vi "多参数标样核查对话框.vi"() -> (2 "确认":bool, 3 "输出参数":T1)   [LabVIEW 2016, in "斯坦道仪器.lvlib"]
panel:
  in  "浊度":bool
  in  "电导率":bool
  in  "pH":bool
  in  "DO":bool
  in  "水温":bool
  in  "组数":dbl=3.0
  in  "取消":bool
  in  "确定":bool
  # "请输入启动参数"
  # "保存组数"
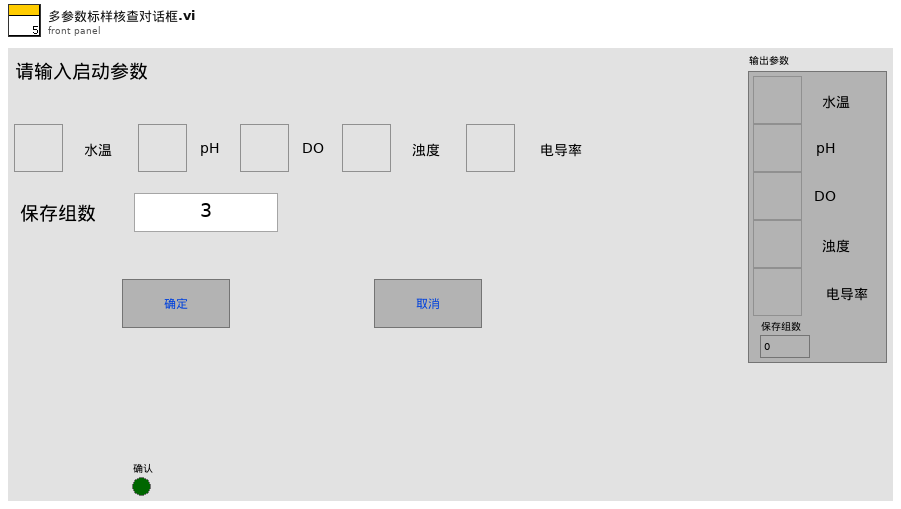
[diagram p1: front panel]
types:
  T1 = cluster{"水温":bool, "pH":bool, "DO":bool, "浊度":bool, "电导率":bool, "保存组数":dbl}
  T2 = cluster{"水温":bool, "pH":bool, "DO":bool, "浊度":bool, "电导率":bool, "组数":dbl}
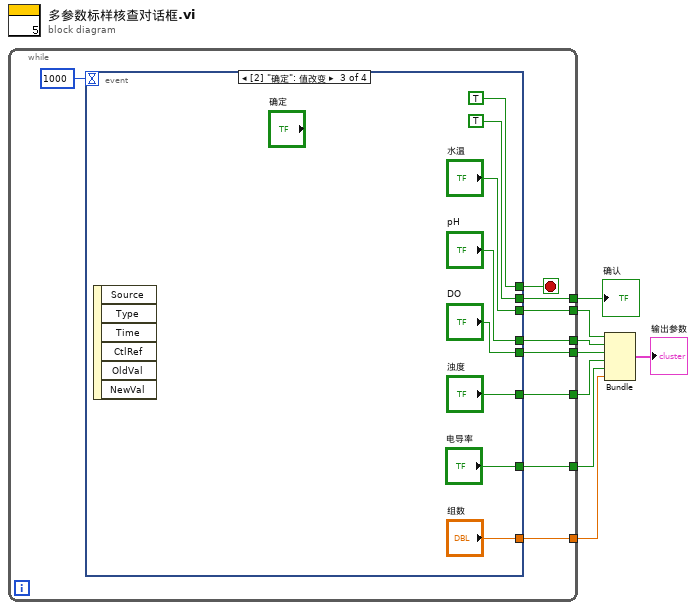
[diagram p0: block diagram]
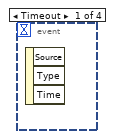
[diagram p2: hidden frame]
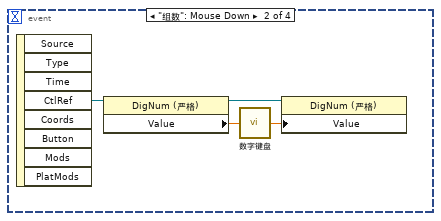
[diagram p3: hidden frame]
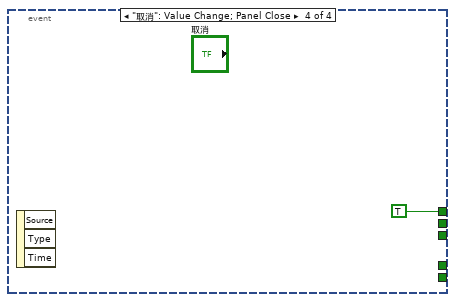
[diagram p4: hidden frame]
diagram:
  n1 = while {
    tunnel: [w15] -> w8
    tunnel: [w14] -> w7
    tunnel: [w13] -> w6
    tunnel: [w12] -> w1
    tunnel: [w11] -> w2
    tunnel: [w10] -> w4
    tunnel: [w9] -> w5
    stop <- w17 stop-if-true
    n2 = event shown="[2] \"确定\": 值改变" {
      selector: _ -> [_ _ _ _]
      dyn-events: _ -> [_ _ _ _]
      timeout: 1000 -> [_ _ _ _]
      tunnel: [_ _ TRUE TRUE] -> w17
      tunnel: [_ _ TRUE _] -> w15
      tunnel: [_ _ "水温" _] -> w14
      tunnel: [_ _ "pH" _] -> w13
      tunnel: [_ _ "电导率" _] -> w12
      tunnel: [_ _ "浊度" _] -> w11
      tunnel: [_ _ "组数" _] -> w10
      tunnel: [_ _ "DO" _] -> w9
      event Timeout {
        n3 = event-data() -> ()  [unwired: 1 in, 3 out]
      }
      event "组数": Mouse Down {
        n4 = event-data() -> ("CtlRef"=w21:refnum<vi>)  [unwired: 1 in, 7 out]
        n5 = property class="DigNum (严格)"(reference=w21) -> (reference out=w19:refnum<vi>, "Value"=w20:dbl)  [unwired: 1 in, 1 out]
        n6 = call "数字键盘.vi"("OldNumber"=w20) -> ("NewNumber"=w18:sgl)
        n7 = property class="DigNum (严格)"(reference=w19, "Value"=w18) -> ()  [unwired: 1 in, 2 out]
      }
      event "确定": Value Change {
        n8 = event-data() -> ()  [unwired: 1 in, 6 out]
      }
      event "取消": Value Change; Panel Close {
        n9 = event-data() -> ()  [unwired: 1 in, 3 out]
      }
    }
  }
  "确认" <- w8
  n10 = Bundle("水温"=w7, "pH"=w6, "DO"=w5, "浊度"=w2, "电导率"=w1, "组数"=w4) -> (→"输出参数":T2)  [unwired: 1 in]
